vi "LNLS Control Decode LOCON_BIPOLAR_16BITS.vi"(6 "error in (no error)":errorcluster, 8 "command body":string) -> (0 "error out":errorcluster, 3 "LOCON data":T1[](array[typedef]) {"status" format="%08b"})   [LabVIEW 2011, in "LNLS Control VIs.lvlib"]
uses:
  LNLS Control VIs.lvlib
  Types Definitions/Type LOCON_BIPOLAR_16BITS.ctl
  Type Definitions.lvlib
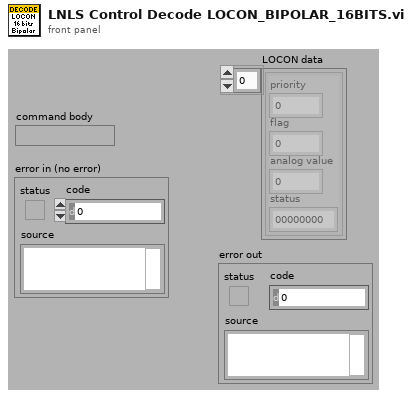
[diagram p1: front panel]
types:
  T1 = typedef "Type Definitions.lvlib/Type LOCON_BIPOLAR_16BITS.ctl" = cluster{"priority":u8, "flag":u8, "analog value":u16, "status":u8}
  T2 = enum16{"big-endian, network order", "native, host order", "little-endian"}
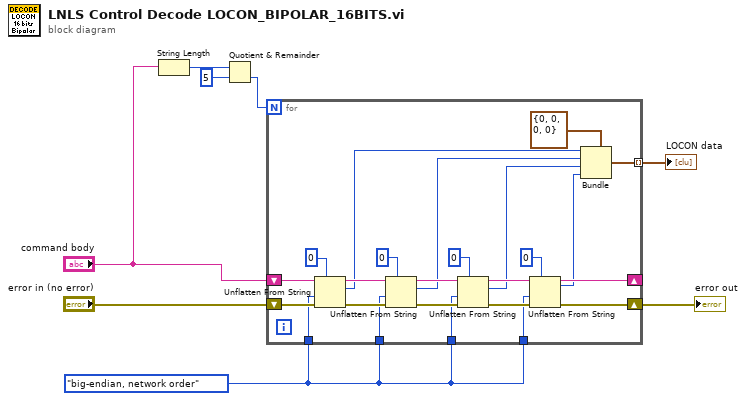
[diagram p0: block diagram]
diagram:
  w6 = T2."big-endian, network order" ("byte order (0:big-endian, network order)")
  n1 = String Length(string="command body") -> (length=w4:i32)
  n2 = Quotient & Remainder(x=w4, y=u8 5) -> (floor(x/y)=w2:i32)  [unwired: 1 out]
  n3 = for {
    N: w2 -> [_]
    shift-right: [w22] -> w8
    shift-left: "error in (no error)" -> [w21]
    shift-right: [w26] -> _
    shift-left: "command body" -> [w32]
    tunnel: [w16] -> w1 mode=indexing
    tunnel: w6 -> [w12]
    tunnel: w6 -> [w11]
    tunnel: w6 -> [w10]
    tunnel: w6 -> [w9]
    n4 = Unflatten From String(type=u8 0 ("priority"), binary string=w32, byte order (0:big-endian, network order)=w9, error in (no error)=w21) -> (rest of the binary string=w29:string, value=w20:u8, error out=w25:errorcluster)  [unwired: 1 in]
    n5 = Unflatten From String(type=u8 0 ("flag"), binary string=w29, byte order (0:big-endian, network order)=w10, error in (no error)=w25) -> (rest of the binary string=w28:string, value=w19:u8, error out=w24:errorcluster)  [unwired: 1 in]
    n6 = Unflatten From String(type=u16 0 ("analog value"), binary string=w28, byte order (0:big-endian, network order)=w11, error in (no error)=w24) -> (rest of the binary string=w27:string, value=w18:u16, error out=w23:errorcluster)  [unwired: 1 in]
    n7 = Unflatten From String(type=u8 0 ("status"), binary string=w27, byte order (0:big-endian, network order)=w12, error in (no error)=w23) -> (rest of the binary string=w26:string, value=w17:u8, error out=w22:errorcluster)  [unwired: 1 in]
    n8 = Bundle(cluster=T1 {"priority"=0, "flag"=0, "analog value"=0, "status"=0}, "priority"=w20, "flag"=w19, "analog value"=w18, "status"=w17) -> (w16:T1)
  }
  "error out" <- w8
  "LOCON data" <- w1
